vi "HumanGlobal.vi"() -> ()   [LabVIEW 2023]
panel:
  in  "ServiceLiftMotorDmd":dbl
  in  "ServiceExtendMotorDmd":dbl
  in  "ServiceRotateMotorDmd":dbl
  out "ServiceMode":bool
  out "CurrentAction":string
  out "Reverse":bool
  out "StateChange":bool
  out "DPadLeft":bool
  out "DPadRight":bool
  out "DPadDown":bool
  out "DPadUp":bool
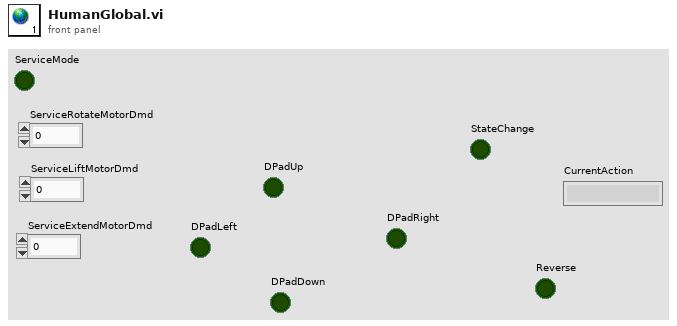
[diagram p1: front panel]
diagram:
